vi "ROSmsg_connectParserTerms.vi"(9 "Previous subVI refnum":refnum<vi>, 11 "New subVI refnum":refnum<vi>) -> (1 "Previous subVI refnum out":refnum<vi>, 3 "New subVI refnum out":refnum<vi>)   [LabVIEW 2016]
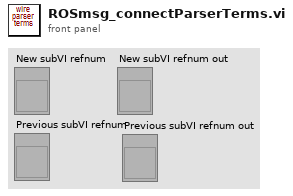
[diagram p1: front panel]
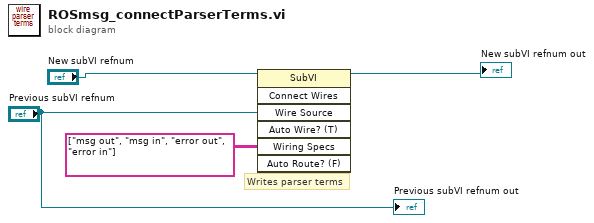
[diagram p0: block diagram]
diagram:
  # "Writes parser terms"
  n1 = invoke class="SubVI" method="Connect Wires"(reference="New subVI refnum", "Wire Source"="Previous subVI refnum", "Wiring Specs"=string[][] [["msg out", "msg in"], ["error out", "error in"]]) -> (reference out=→"New subVI refnum out":refnum<vi>)  [unwired: 4 in, 6 out]
  "Previous subVI refnum out" <- "Previous subVI refnum"
